vi "RefreshSubTreeWithGlyphManager.vi"(8 "error in":errorcluster, 9 "glyph manager":T1, 10 "node information":T3[](array[typedef]), 11 "tree ref in":refnum<vi>) -> (0 "error out":errorcluster, 1 "glyph manager out":T1, 3 "tree ref out":refnum<vi>)   [LabVIEW 2025, in "CEF.lvlib"]
doc: "Updates just a portion of the tree controlCopyright 2017 National Instruments Corporation\n\nLicensed under the Apache License, Version 2.0 (the \"License\"); you may not use this file except in compliance with the License. You may obtain a copy of the License at http://www.apache.org/licenses/LICENSE-2.0\nUnless required by applicable law or agreed to in writing, software distributed under the License is distributed on an \"AS IS\" BASIS, WITHOUT WARRANTIES OR CONDITIONS OF ANY KIND, either express or implied. See the License for the specific language governing permissions and limitations under the License."
uses:
  CEF.lvlib
  Node/Summary.ctl
  glyph manager/glyph manager.ctl
  <vilib>/picture/picture.llb/imagedata.ctl
  Node/CEF_Node.lvclass
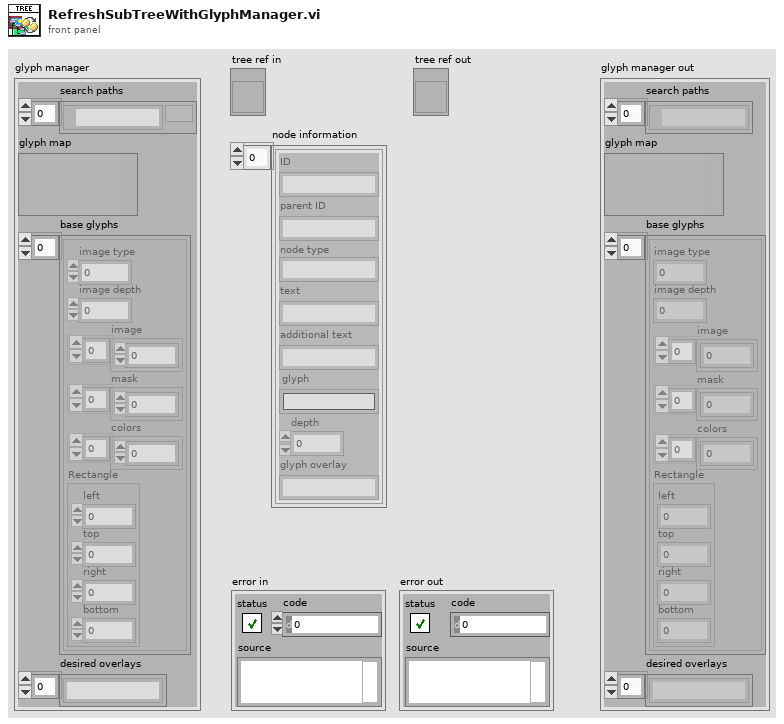
[diagram p1: front panel]
types:
  T1 = typedef "CEF.lvlib/glyph manager.ctl" = cluster{"search paths":path[], "glyph map":variant, "base glyphs":T2[], "desired overlays":string[]}
  T2 = typedef "imagedata.ctl" = cluster{"image type":i32, "image depth":i32, "image":u8[], "mask":u8[], "colors":u32[], "Rectangle":cluster{"left":i16, "top":i16, "right":i16, "bottom":i16}}
  T3 = typedef "CEF.lvlib/CEF_Node.lvclass/Summary.ctl" = cluster{"ID":string, "parent ID":string, "node type":string, "text":string, "additional text":string, "glyph":string, "depth":i32, "glyph overlay":string}
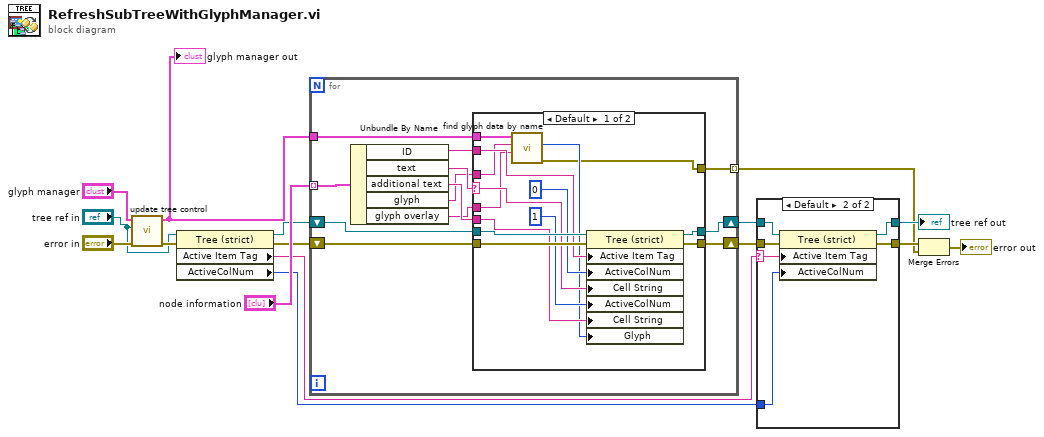
[diagram p0: block diagram]
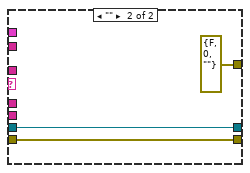
[diagram p3: hidden frame]
diagram:
  n1 = call "update tree control.vi"("error in"="error in", "tree reference"="tree ref in", "glyph manager in"="glyph manager") -> ("error out"=w4:errorcluster, "glyph manager out"=w2:T1)  [unwired: 7 in]
  "glyph manager out" <- w2
  n2 = property class="Tree (strict)"(reference="tree ref in", error in=w4) -> (reference out=w15:refnum<vi>, error out=w13:errorcluster, "Active Item Tag"=w9:string, "ActiveColNum"=w8:i32)
  n3 = for {
    shift-right: [w27] -> w10
    shift-left: w13 -> [w26]
    tunnel: "node information" -> [w28] mode=indexing
    shift-right: [w24] -> w11
    shift-left: w15 -> [w23]
    tunnel: [w19] -> w6 mode=indexing
    tunnel: w2 -> [w17]
    n4 = Unbundle By Name(w28) -> ("ID"=w22:string, "text"=w25:string, "additional text"=w21:string, "glyph"=w20:string, "glyph overlay"=w18:string)
    n5 = case shown="Default" w25 {
      selector: w25 -> [w36 _]
      tunnel: [w39 w45] -> w27
      tunnel: w26 -> [w40 w45]
      tunnel: [w41 w44] -> w24
      tunnel: w23 -> [w42 w44]
      tunnel: w22 -> [w38 _]
      tunnel: w21 -> [w34 _]
      tunnel: w20 -> [w33 _]
      tunnel: [w29 errorcluster {"status"=FALSE, "code"=0, "source"=""} ("error out")] -> w19
      tunnel: w18 -> [w32 _]
      tunnel: w17 -> [w31 _]
      frame Default {
        n6 = call "find glyph data by name.vi"("overlay"=w32, "name"=w33, "glyph manager in"=w31) -> ("error out"=w29:errorcluster, "symbol index"=w30:i32)  [unwired: 5 in, 2 out]
        n7 = property class="Tree (strict)"(reference=w42, error in=w40, "Active Item Tag"=w38, "ActiveColNum"=0 ("Active Cell:Active Column Number"), "Cell String"=w36, "ActiveColNum"=1 ("Active Cell:Active Column Number"), "Cell String"=w34, "Glyph"=w30) -> (reference out=w41:refnum<vi>, error out=w39:errorcluster)
      }
      frame "" {
      }
    }
  }
  n8 = case shown="Default" w9 {
    selector: w9 -> [_ w48]
    tunnel: [w47 w53] -> w12
    tunnel: w11 -> [w47 w52]
    tunnel: w10 -> [w46 w51]
    tunnel: w8 -> [_ w50]
    tunnel: [w46 w49] -> w7
    frame "" {
    }
    frame Default {
      n9 = property class="Tree (strict)"(reference=w52, error in=w51, "Active Item Tag"=w48, "ActiveColNum"=w50) -> (reference out=w53:refnum<vi>, error out=w49:errorcluster)
    }
  }
  "tree ref out" <- w12
  n10 = Merge Errors(w7, w6) -> (→"error out":errorcluster)
